vi "_DataPluginInstallAndRefresh.vi"(6 "Install?":bool, 8 "error in":errorcluster, 9 "Item Names":string[][](array[string]), 10 "Value":i32[](array[numeric]), 11 "DataPlugin Info":T1[](array[typedef])) -> (0 "error out":errorcluster, 1 "Results":string[][](array[string]), 2 "Item Names out":string[][](array[string]), 3 "DataPlugin information out":T1[](array[typedef]), 4 "Indices":i32[](array[numeric]))   [LabVIEW 2017]
uses:
  <vilib>/Platform/storage/utility/DataPluginSynchronization/_DataPluginInfo.ctl
  <vilib>/Platform/storage/utility/DataPluginSynchronization/_localizeDataPluginMessageEnum.ctl
  <vilib>/Platform/storage/utility/Install DataPlugin by Name.vi
panel:
  out "Boolean":bool
  out "String":string="Downloading the installer and installing the DataPlugins on the computer"
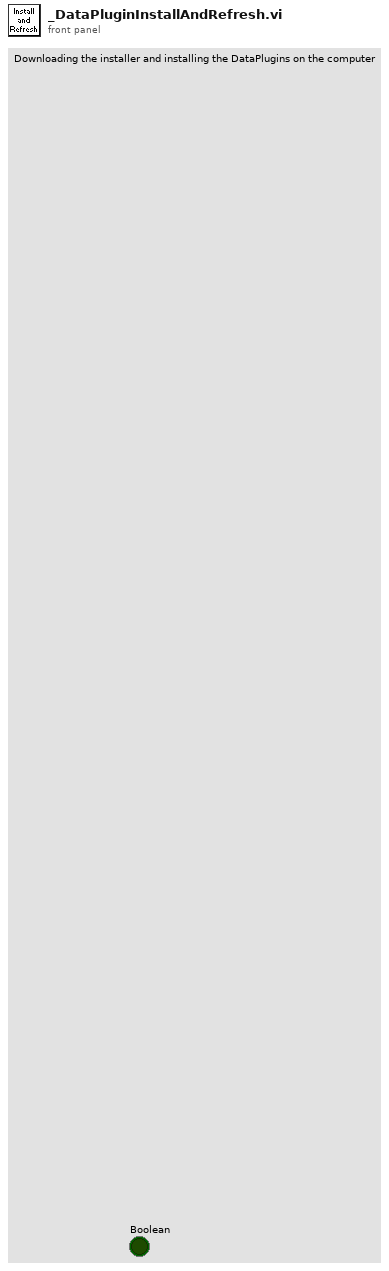
[diagram p1: front panel]
types:
  T1 = typedef "_DataPluginInfo.ctl" = cluster{"name":string, "status":u32, "extensions":string[], "description":string, "url":string, "lastExportTime":i64, "type":string, "version":string, "exist":bool, "current version":string, "model":string}
  T2 = typedef "_localizeDataPluginMessageEnum.ctl" = enum16{"Installed", "Not Installed", "Updates Available", "Latest version:", "Double click the \"Description\" cell.", "Install/Update DataPlugins", "Offline: ", "Please ensure that your network connection is working.", "No DataPlugins can be updated.", "Loading DataPlugins from ni.com/dataplugins", "Acquiring and installing ", "Install", "Update", "Succeed", "Failed", " Installation successful.", "Include *. to search for a file extension", "Current version:", " Installation failed.", "Installing update", "Update successful.", "Update failed.", "Updated", "Failed to update DataPlugins."}
  T3 = typedef "usiPluginInformation.ctl" = cluster{"name":string, "version":string, "type":string, "read-only?":bool, "extensions":string[]}
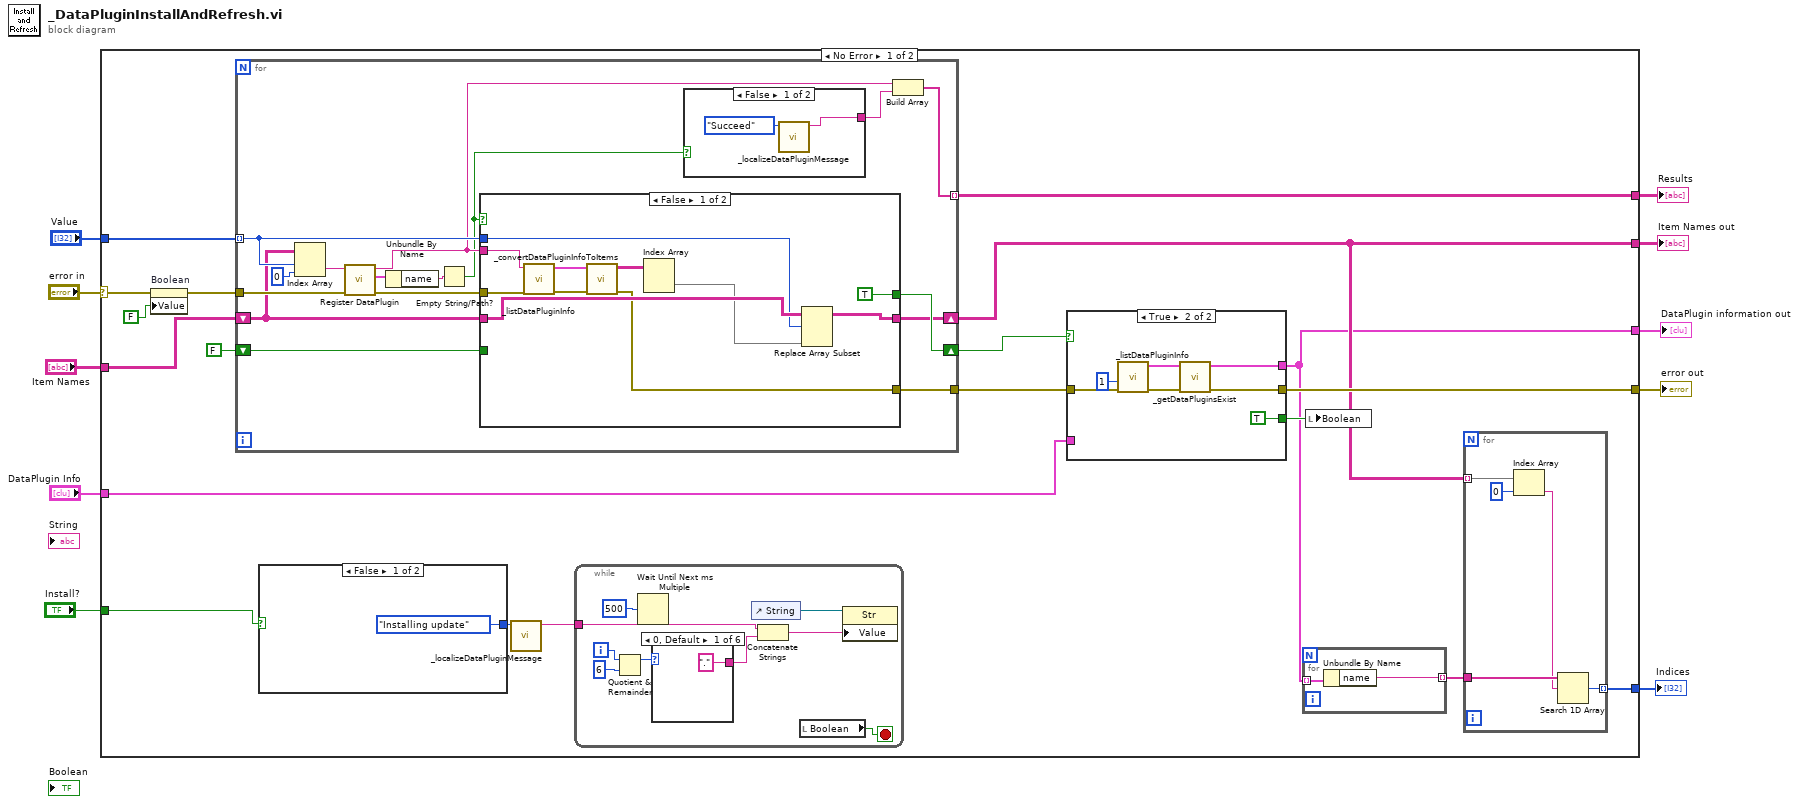
[diagram p0: block diagram]
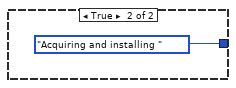
[diagram p2: hidden frame]
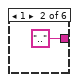
[diagram p3: hidden frame]
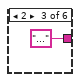
[diagram p4: hidden frame]
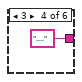
[diagram p5: hidden frame]
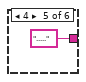
[diagram p6: hidden frame]
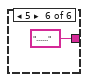
[diagram p7: hidden frame]
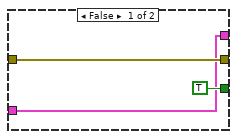
[diagram p8: hidden frame]
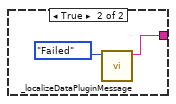
[diagram p9: hidden frame]
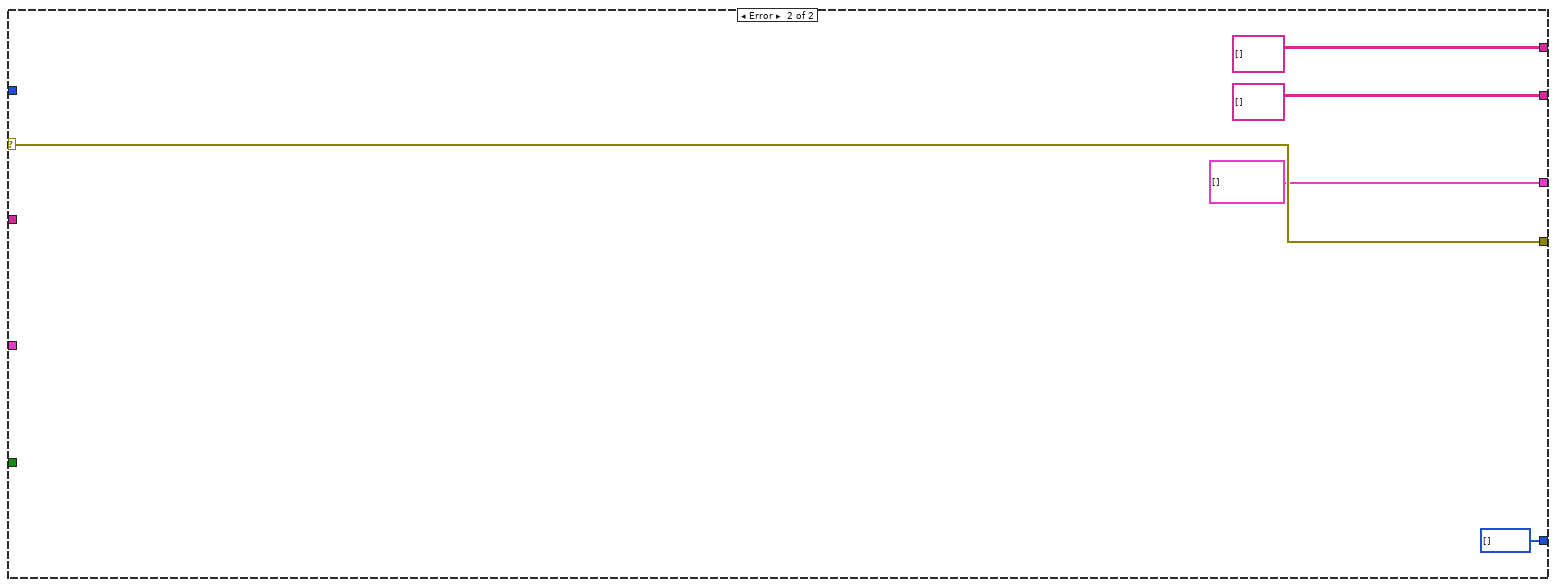
[diagram p11: hidden frame]
diagram:
  n1 = case shown="No Error" "error in" {
    selector: "error in" -> [w18 w102]
    tunnel: "Value" -> [w29 _]
    tunnel: [w28 w102] -> w9
    tunnel: "Item Names" -> [w27 _]
    tunnel: [w13 T1[] [] ("DataPlugin information")] -> w7
    tunnel: [w14 string[][] [] ("Item Names")] -> w6
    tunnel: [w20 string[][] []] -> w5
    tunnel: "DataPlugin Info" -> [w19 _]
    tunnel: "Install?" -> [w15 _]
    tunnel: [w11 i32[] []] -> w1
    frame No Error {
      n2 = property on="Boolean" class="Bool (strict)"(error in=w18, "Value"=FALSE ("Boolean")) -> (error out=w21:errorcluster)  [unwired: 1 in, 1 out]
      n3 = for {
        tunnel: w29 -> [w74] mode=indexing
        shift-right: [w77] -> w24
        shift-left: FALSE ("refresh") -> [w78]
        tunnel: w21 -> [w75]
        tunnel: [w70] -> w25
        shift-right: [w73] -> w14
        shift-left: w27 -> [w72]
        tunnel: [w67] -> w20 mode=indexing
        n4 = Index Array(array=w72, index (row)=w74, index (col)=0 ("disabled index (col)")) -> (element=w76:string)
        n5 = call-poly <vilib>:"Register DataPlugin.vi"("error in (no error)"=w75, "DataPlugin name"=w76) -> ("error out"=w71:errorcluster, "DataPlugin information"=w66:T3, "DataPlugin name out"=w69:string)  [unwired: 7 in]
        n6 = Unbundle By Name(w66) -> ("name"=w64:string)
        n7 = Empty String/Path?(string/path=w64) -> (empty?=w65:bool)
        n8 = case shown="False" w65 {
          tunnel: w69 -> [w89 _]
          tunnel: [w93 w96] -> w73
          tunnel: [TRUE ("refresh") w97] -> w77
          tunnel: w78 -> [_ w97]
          tunnel: w72 -> [w92 w96]
          tunnel: w74 -> [w91 _]
          tunnel: w71 -> [w90 w95]
          tunnel: [w84 w95] -> w70
          frame False {
            n9 = call <vilib>:"_listDataPluginInfo.vi"("error in (no error)"=w90, "DataPlugin name"=w89) -> ("error out"=w87:errorcluster, "DataPlugin information"=w88:T1[])  [unwired: 8 in]
            n10 = call <vilib>:"_convertDataPluginInfoToItems.vi"("error in (no error)"=w87, "DataPlugin information"=w88) -> ("error out"=w84:errorcluster, "Items"=w86:string[][])  [unwired: 8 in]
            n11 = Index Array(array=w86) -> (element=w85:string[])  [unwired: 2 in]
            n12 = Replace Array Subset(array=w92, new element=w85, index (row)=w91) -> (w93:string[][])  [unwired: 1 in]
          }
          frame True {
          }
        }
        n13 = case shown="False" w65 {
          tunnel: [w81 w83] -> w68
          frame False {
            n14 = call <vilib>:"_localizeDataPluginMessage.vi"("message in"=_localizeDataPluginMessageEnum."Succeed") -> ("message out"=w81:string)  [unwired: 10 in]
          }
          frame True {
            n15 = call <vilib>:"_localizeDataPluginMessage.vi"("message in"=_localizeDataPluginMessageEnum."Failed") -> ("message out"=w83:string)  [unwired: 10 in]
          }
        }
        n16 = Build Array(w69, w68) -> (w67:string[])
      }
      n17 = case shown="False" w15 {
        tunnel: [_localizeDataPluginMessageEnum."Installing update" ("message in") _localizeDataPluginMessageEnum."Acquiring and installing " ("message in")] -> w17
        frame False {
        }
        frame True {
        }
      }
      n18 = call <vilib>:"_localizeDataPluginMessage.vi"("message in"=w17) -> ("message out"=w16:string)  [unwired: 10 in]
      n19 = while {
        tunnel: w16 -> [w40]
        i -> [w47]
        stop <- w41 stop-if-true
        n20 = Quotient & Remainder(x=w47, y=6) -> (x-y*floor(x/y)=w44:i32)  [unwired: 1 out]
        n21 = Wait Until Next ms Multiple(millisecond multiple=u32 500) -> ()  [unwired: 1 out]
        n22 = case shown="0, Default" w44 {
          tunnel: ["." ("y") ".." ("y") "..." ("y") "...." ("y") "....." ("y") "......" ("y")] -> w45
          frame 0, Default {
          }
          frame 1 {
          }
          frame 2 {
          }
          frame 3 {
          }
          frame 4 {
          }
          frame 5 {
          }
        }
        n23 = control-ref of="String"() -> (w42:refnum<vi>)
        n24 = Concatenate Strings(w40, w45) -> (w39:string)
        n25 = local read "Boolean"() -> (w41:bool)
        n26 = property class="Str"(reference=w42, "Value"=w39) -> ()  [unwired: 1 in, 2 out]
      }
      n27 = case shown="True" w24 {
        tunnel: [w56 w57] -> w28
        tunnel: w19 -> [w54 _]
        tunnel: w25 -> [w56 w62]
        tunnel: [TRUE ("refresh") TRUE ("refresh")] -> w23
        tunnel: [w54 w59] -> w13
        frame False {
        }
        frame True {
          n28 = call <vilib>:"_listDataPluginInfo.vi"("error in (no error)"=w62, "source"=u32 1) -> ("error out"=w58:errorcluster, "DataPlugin information"=w60:T1[])  [unwired: 8 in]
          n29 = call <vilib>:"_getDataPluginsExist.vi"("error in (no error)"=w58, "DataPlugin information in"=w60) -> ("error out"=w57:errorcluster, "DataPlugin information out"=w59:T1[])  [unwired: 8 in]
        }
      }
      n30 = for {
        tunnel: w13 -> [w31] mode=indexing
        tunnel: [w30] -> w12 mode=indexing
        n31 = Unbundle By Name(w31) -> ("name"=w30:string)
      }
      n32 = local write "Boolean"(w23) -> ()
      n33 = for {
        tunnel: w14 -> [w36] mode=indexing
        tunnel: w12 -> [w34]
        tunnel: [w33] -> w11 mode=indexing
        n34 = Index Array(array=w36, index=0) -> (element=w32:string)
        n35 = Search 1D Array(1D array=w34, element=w32) -> (index of element=w33:i32)  [unwired: 1 in]
      }
    }
    frame Error {
    }
  }
  "error out" <- w9
  "Item Names out" <- w6
  "DataPlugin information out" <- w7
  "Results" <- w5
  "Indices" <- w1
